vi "Settings_to_Queue.vi"(0 "File path user settings":path) -> ()   [LabVIEW 2012]
uses:
  <vilib>/Utility/config.llb/Read Key (I32).vi
  <vilib>/Utility/config.llb/Read Key (String).vi
  <vilib>/Utility/config.llb/Read Key (Boolean).vi
  <vilib>/Utility/config.llb/Read Key (Double).vi
  <vilib>/Utility/config.llb/NI_LVConfig.lvlib
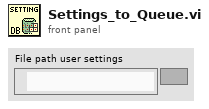
[diagram p1: front panel]
types:
  T1 = typedef "NI_LVConfig.lvlib/Config Data RefNum.ctl" = refnum<k1>
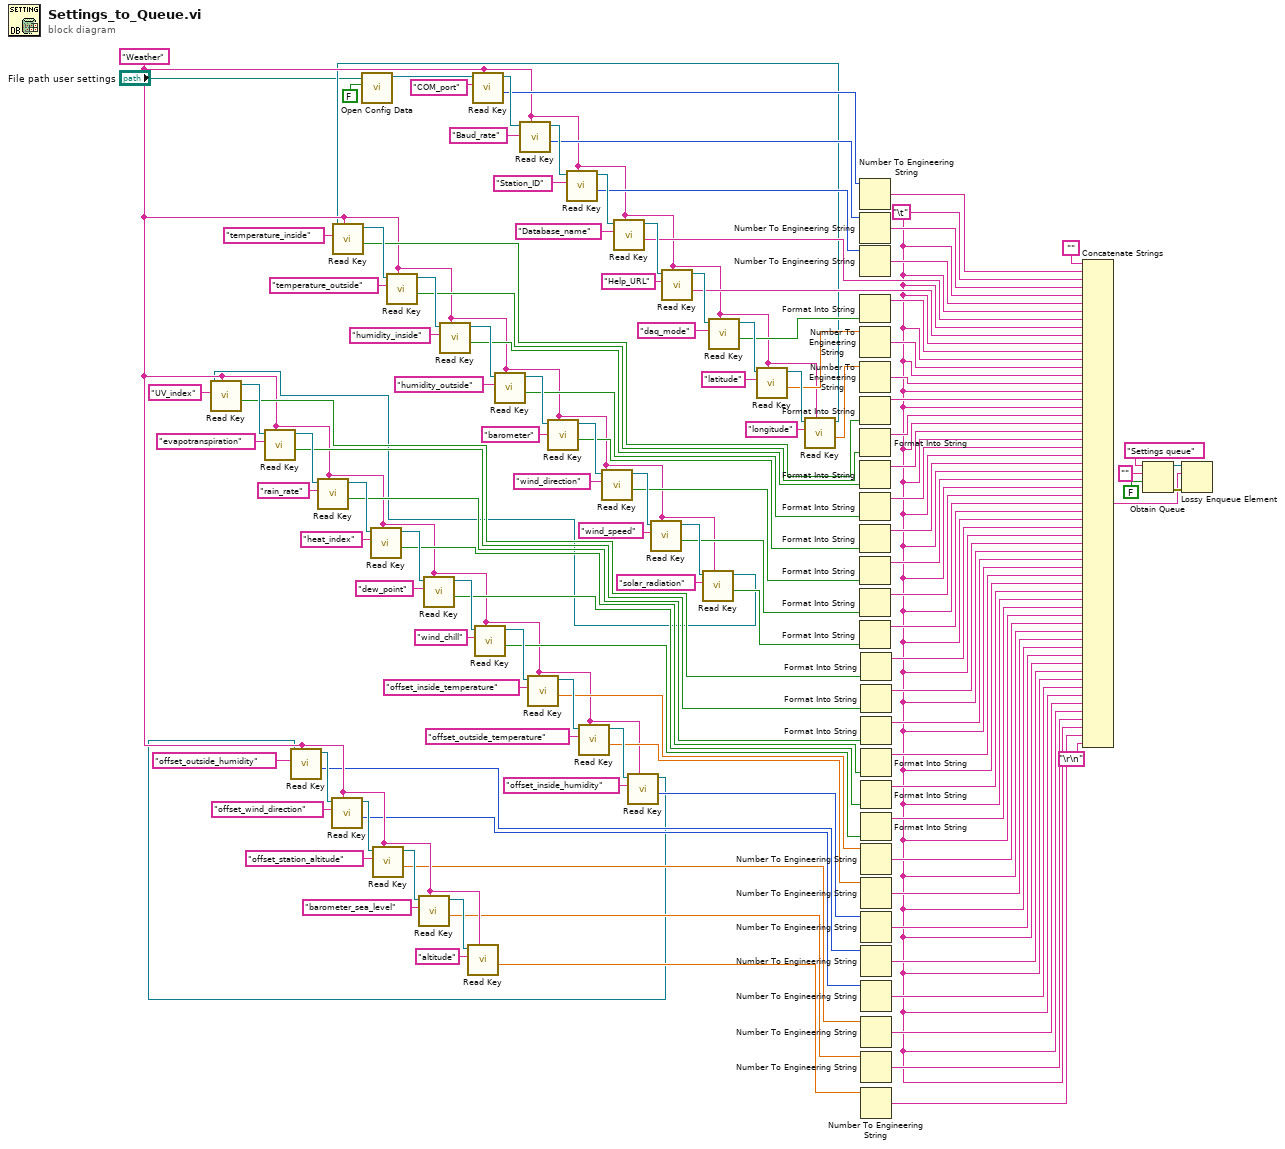
[diagram p0: block diagram]
diagram:
  w7 = "\t"
  w18 = "Weather" ("section")
  n1 = call <vilib>:"Open Config Data.vi"("create file if necessary (T)"=FALSE, "configuration file path"="File path user settings") -> ("refnum"=w121:T1)  [unwired: 7 in, 2 out]
  n2 = call-poly <vilib>:"Read Key.vi"("section"=w18, "key"="COM_port", "refnum"=w121) -> ("value"=w74:i32, "refnum out"=w120:T1)  [unwired: 5 in, 2 out]
  n3 = call-poly <vilib>:"Read Key.vi"("section"=w18, "key"="Baud_rate", "refnum"=w120) -> ("value"=w72:i32, "refnum out"=w87:T1)  [unwired: 5 in, 2 out]
  n4 = call-poly <vilib>:"Read Key.vi"("section"=w18, "key"="Station_ID", "refnum"=w87) -> ("value"=w71:i32, "refnum out"=w86:T1)  [unwired: 5 in, 2 out]
  n5 = call-poly <vilib>:"Read Key.vi"("section"=w18, "key"="Database_name" ("Key name"), "refnum"=w86) -> ("value"=w70:string, "refnum out"=w85:T1)  [unwired: 5 in, 2 out]
  n6 = call-poly <vilib>:"Read Key.vi"("section"=w18, "key"="Help_URL" ("Key name"), "refnum"=w85) -> ("value"=w69:string, "refnum out"=w84:T1)  [unwired: 5 in, 2 out]
  n7 = call-poly <vilib>:"Read Key.vi"("section"=w18, "key"="daq_mode", "refnum"=w84) -> ("value"=w67:bool, "refnum out"=w83:T1)  [unwired: 5 in, 2 out]
  n8 = call-poly <vilib>:"Read Key.vi"("section"=w18, "key"="latitude", "refnum"=w83) -> ("value"=w66:dbl, "refnum out"=w82:T1)  [unwired: 5 in, 2 out]
  n9 = call-poly <vilib>:"Read Key.vi"("section"=w18, "key"="longitude", "refnum"=w82) -> ("value"=w65:dbl, "refnum out"=w4:T1)  [unwired: 5 in, 2 out]
  n10 = call-poly <vilib>:"Read Key.vi"("section"=w18, "key"="temperature_inside", "refnum"=w4) -> ("value"=w53:bool, "refnum out"=w81:T1)  [unwired: 5 in, 2 out]
  n11 = call-poly <vilib>:"Read Key.vi"("section"=w18, "key"="temperature_outside", "refnum"=w81) -> ("value"=w52:bool, "refnum out"=w80:T1)  [unwired: 5 in, 2 out]
  n12 = call-poly <vilib>:"Read Key.vi"("section"=w18, "key"="humidity_inside", "refnum"=w80) -> ("value"=w50:bool, "refnum out"=w79:T1)  [unwired: 5 in, 2 out]
  n13 = call-poly <vilib>:"Read Key.vi"("section"=w18, "key"="humidity_outside", "refnum"=w79) -> ("value"=w57:bool, "refnum out"=w78:T1)  [unwired: 5 in, 2 out]
  n14 = call-poly <vilib>:"Read Key.vi"("section"=w18, "key"="barometer", "refnum"=w78) -> ("value"=w51:bool, "refnum out"=w77:T1)  [unwired: 5 in, 2 out]
  n15 = call-poly <vilib>:"Read Key.vi"("section"=w18, "key"="wind_direction", "refnum"=w77) -> ("value"=w56:bool, "refnum out"=w76:T1)  [unwired: 5 in, 2 out]
  n16 = call-poly <vilib>:"Read Key.vi"("section"=w18, "key"="wind_speed", "refnum"=w76) -> ("value"=w54:bool, "refnum out"=w75:T1)  [unwired: 5 in, 2 out]
  n17 = call-poly <vilib>:"Read Key.vi"("section"=w18, "key"="solar_radiation", "refnum"=w75) -> ("value"=w55:bool, "refnum out"=w3:T1)  [unwired: 5 in, 2 out]
  n18 = call-poly <vilib>:"Read Key.vi"("section"=w18, "key"="UV_index", "refnum"=w3) -> ("value"=w37:bool, "refnum out"=w42:T1)  [unwired: 5 in, 2 out]
  n19 = call-poly <vilib>:"Read Key.vi"("section"=w18, "key"="evapotranspiration", "refnum"=w42) -> ("value"=w36:bool, "refnum out"=w41:T1)  [unwired: 5 in, 2 out]
  n20 = call-poly <vilib>:"Read Key.vi"("section"=w18, "key"="rain_rate", "refnum"=w41) -> ("value"=w35:bool, "refnum out"=w40:T1)  [unwired: 5 in, 2 out]
  n21 = call-poly <vilib>:"Read Key.vi"("section"=w18, "key"="heat_index", "refnum"=w40) -> ("value"=w31:bool, "refnum out"=w39:T1)  [unwired: 5 in, 2 out]
  n22 = call-poly <vilib>:"Read Key.vi"("section"=w18, "key"="dew_point", "refnum"=w39) -> ("value"=w30:bool, "refnum out"=w38:T1)  [unwired: 5 in, 2 out]
  n23 = call-poly <vilib>:"Read Key.vi"("section"=w18, "key"="wind_chill", "refnum"=w38) -> ("value"=w29:bool, "refnum out"=w34:T1)  [unwired: 5 in, 2 out]
  n24 = call-poly <vilib>:"Read Key.vi"("section"=w18, "key"="offset_inside_temperature", "refnum"=w34) -> ("value"=w28:dbl, "refnum out"=w33:T1)  [unwired: 5 in, 2 out]
  n25 = call-poly <vilib>:"Read Key.vi"("section"=w18, "key"="offset_outside_temperature", "refnum"=w33) -> ("value"=w27:dbl, "refnum out"=w32:T1)  [unwired: 5 in, 2 out]
  n26 = call-poly <vilib>:"Read Key.vi"("section"=w18, "key"="offset_inside_humidity", "refnum"=w32) -> ("value"=w26:i32, "refnum out"=w2:T1)  [unwired: 5 in, 2 out]
  n27 = call-poly <vilib>:"Read Key.vi"("section"=w18, "key"="offset_outside_humidity", "refnum"=w2) -> ("value"=w17:i32, "refnum out"=w22:T1)  [unwired: 5 in, 2 out]
  n28 = call-poly <vilib>:"Read Key.vi"("section"=w18, "key"="offset_wind_direction", "refnum"=w22) -> ("value"=w16:i32, "refnum out"=w21:T1)  [unwired: 5 in, 2 out]
  n29 = call-poly <vilib>:"Read Key.vi"("section"=w18, "key"="offset_station_altitude", "refnum"=w21) -> ("value"=w15:dbl, "refnum out"=w20:T1)  [unwired: 5 in, 2 out]
  n30 = call-poly <vilib>:"Read Key.vi"("section"=w18, "key"="barometer_sea_level", "refnum"=w20) -> ("value"=w14:dbl, "refnum out"=w19:T1)  [unwired: 5 in, 2 out]
  n31 = call-poly <vilib>:"Read Key.vi"("section"=w18, "key"="altitude", "refnum"=w19) -> ("value"=w13:dbl)  [unwired: 5 in, 3 out]
  n32 = Number To Engineering String(4:w74) -> (0:w73:string)  [unwired: 3 out]
  n33 = Number To Engineering String(4:w72) -> (0:w89:string)  [unwired: 3 out]
  n34 = Number To Engineering String(4:w71) -> (0:w88:string)  [unwired: 3 out]
  n35 = Format Into String(w67) -> (resulting string=w68:string)  [unwired: 3 in, 1 out]
  n36 = Number To Engineering String(4:w66) -> (0:w91:string)  [unwired: 3 out]
  n37 = Number To Engineering String(4:w65) -> (0:w90:string)  [unwired: 3 out]
  n38 = Format Into String(w53) -> (resulting string=w64:string)  [unwired: 3 in, 1 out]
  n39 = Format Into String(w52) -> (resulting string=w63:string)  [unwired: 3 in, 1 out]
  n40 = Format Into String(w50) -> (resulting string=w58:string)  [unwired: 3 in, 1 out]
  n41 = Format Into String(w57) -> (resulting string=w59:string)  [unwired: 3 in, 1 out]
  n42 = Format Into String(w51) -> (resulting string=w60:string)  [unwired: 3 in, 1 out]
  n43 = Format Into String(w56) -> (resulting string=w61:string)  [unwired: 3 in, 1 out]
  n44 = Format Into String(w54) -> (resulting string=w62:string)  [unwired: 3 in, 1 out]
  n45 = Format Into String(w55) -> (resulting string=w49:string)  [unwired: 3 in, 1 out]
  n46 = Format Into String(w37) -> (resulting string=w48:string)  [unwired: 3 in, 1 out]
  n47 = Format Into String(w36) -> (resulting string=w47:string)  [unwired: 3 in, 1 out]
  n48 = Format Into String(w35) -> (resulting string=w46:string)  [unwired: 3 in, 1 out]
  n49 = Format Into String(w31) -> (resulting string=w45:string)  [unwired: 3 in, 1 out]
  n50 = Format Into String(w30) -> (resulting string=w44:string)  [unwired: 3 in, 1 out]
  n51 = Format Into String(w29) -> (resulting string=w43:string)  [unwired: 3 in, 1 out]
  n52 = Number To Engineering String(4:w28) -> (0:w25:string)  [unwired: 3 out]
  n53 = Number To Engineering String(4:w27) -> (0:w24:string)  [unwired: 3 out]
  n54 = Number To Engineering String(4:w26) -> (0:w23:string)  [unwired: 3 out]
  n55 = Number To Engineering String(4:w17) -> (0:w12:string)  [unwired: 3 out]
  n56 = Number To Engineering String(4:w16) -> (0:w11:string)  [unwired: 3 out]
  n57 = Number To Engineering String(4:w15) -> (0:w10:string)  [unwired: 3 out]
  n58 = Number To Engineering String(4:w14) -> (0:w9:string)  [unwired: 3 out]
  n59 = Number To Engineering String(4:w13) -> (0:w8:string)  [unwired: 3 out]
  n60 = Concatenate Strings("", w73, w7, w89, w7, w88, w7, w70, w7, w69, w7, w68, w7, w91, w7, w90, w7, w64, w7, w63, w7, w58, w7, w59, w7, w60, w7, w61, w7, w62, w7, w49, w7, w48, w7, w47, w7, w46, w7, w45, w7, w44, w7, w43, w7, w25, w7, w24, w7, w23, w7, w12, w7, w11, w7, w10, w7, w9, w7, w8, "\r\n") -> (w6:string)
  n61 = Obtain Queue(name (unnamed)="Settings queue", element data type="" ("name (unnamed)"), create if not found? (T)=FALSE) -> (queue out=w94:refnum<queue>, error out=w93:errorcluster)  [unwired: 2 in, 1 out]
  n62 = Lossy Enqueue Element(queue=w94, element=w6, error in (no error)=w93) -> ()  [unwired: 4 out]
